vi "Convert Device Units to Speed Units (Polymorphic).vi"   [LabVIEW 2013, in "Zaber A Series.lvlib"]
doc: "Helper to convert device-specific speed units to standard units of speed.\n\nSelect a unit to convert to and enter a speed measurement from a Zaber device. The measurement will be converted to the selected units.\n\nIf you select a unit other than device speed units, you must also provide the Microstep Size conversion factor from microsteps to micrometers (for linear stages) or degrees (for rotary stages), which can be found in your device manual."
uses:
  Zaber A Series.lvlib
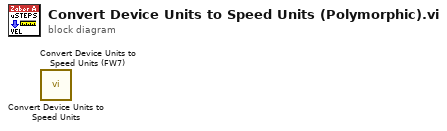
[diagram p0: block diagram]
diagram:
  n1 = call "Convert Device Units to Speed Units.vi"() -> ()  [unwired: 11 in, 1 out]
  n2 = call "Convert Device Units to Speed Units (FW7).vi"() -> ()  [unwired: 11 in, 1 out]
